vi "Periodic Tasks.vi"(8 "error in":errorcluster) -> ()   [LabVIEW 2014]
doc: "This VI runs in parallel to other tasks. It can contain as many user-defined periodic loops as you need. These can carry out PID or other sorts of timed response."
uses:
  <vilib>/Rock Robotics/WPI/Solenoid/WPI_SolenoidValue.ctl
  <vilib>/Rock Robotics/WPI/Joystick/WPI_JoystickGetSetRefNum.vi
  <vilib>/Rock Robotics/WPI/RobotDrive/WPI_RobotDriveGetSetRefNum.vi
  <vilib>/Rock Robotics/WPI/Solenoid/WPI_SolenoidSetEnum.vi
  <vilib>/Rock Robotics/WPI/Ultrasonic/WPI_UltrasonicRangeUnits.ctl
  <vilib>/Rock Robotics/WPI/Ultrasonic/WPI_SonarMB1010AnalogRefNum Registry Get.vi
panel:
  out "AVG Gyro Angle":dbl
  out "Gyro Angle 2":dbl
  out "error out":errorcluster
  out "Ultrasonic":i16
  out "USD Encoder":dbl
  out "limit switch":bool
  out "XY Graph 2":cluster{"Y":dbl[], "Y":dbl[]}[](graph)
  out "Accelerations":T1
  out "optical":bool
  out "potentiometer":dbl
  out "Gyro Angle":dbl
  out "Grayhill Encoder":dbl
  out "PDP voltage (V) IN":dbl
  in  "Value 2":T2
  in  "Value":T2
  in  "Output":dbl
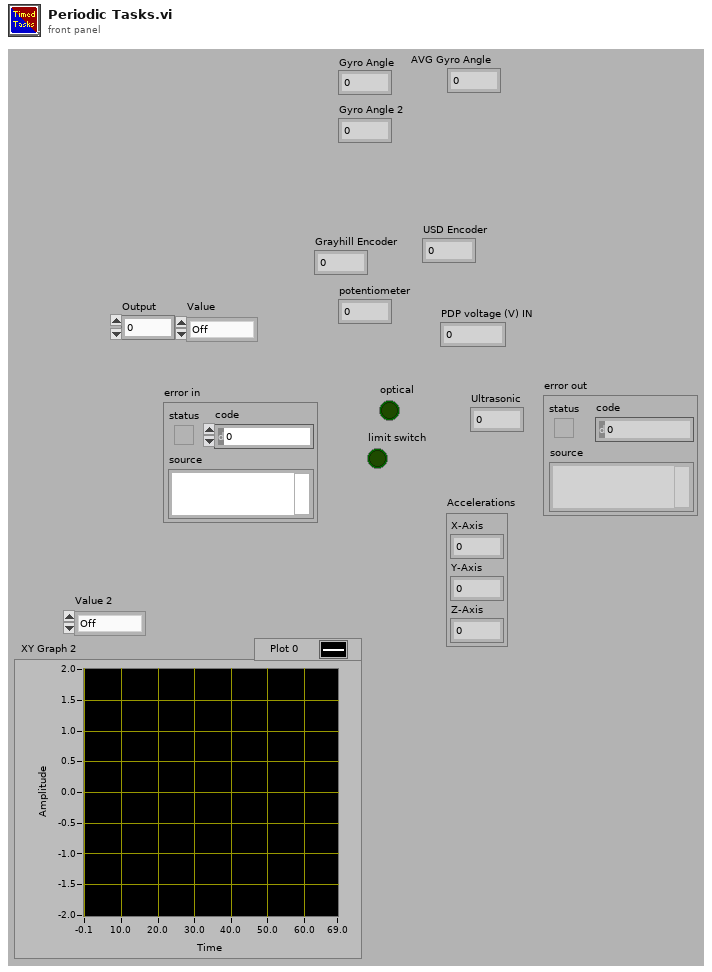
[diagram p1: front panel]
types:
  T1 = cluster{"X-Axis":dbl, "Y-Axis":dbl, "Z-Axis":dbl}
  T2 = typedef "WPI_SolenoidValue.ctl" = enum16{"Off", "On", "Forward", "Reverse"}
  T3 = typedef "WPI_CameraDevRef.ctl" = cluster{"Camera Address":string, "CameraStatus":errorcluster}
  T4 = typedef "WPI_JoystickDevRef.ctl" = cluster{"Device":T5}
  T5 = typedef "WPI_JoystickDeviceEnum.ctl" = enum16{"USB 0", "USB 1", "USB 2", "USB 3", "USB 4", "USB 5"}
  T6 = typedef "WPI_RobotDriveDevRef.ctl" = cluster{"DevStatus":errorcluster, "Motors[]":T7[], "Square Inputs":bool, "Max Output":dbl}
  T7 = typedef "WPI_MotorControlDeviceRef.ctl" = cluster{"DeviceStatus":errorcluster, "Type":T8, "PWM":cluster{"Controller":T9, "PWM Channel":T10, "DeadBand":T11}, "CAN":cluster{"Device Number":u8, "Control Mode":T12, "Semaphore":T13, "Max Vout":dbl, "TalonSRX Control Mode":T14}, "Invert":bool, "TransformRef":T15, "InvTransformRef":T15}
  T8 = typedef "WPI_MotorControlType.ctl" = enum16{"PWM", "CAN", "CANTalonSRX"}
  T9 = typedef "FPGA_TypedefDigitalModule.ctl" = enum16{"Controller 1"}
  T10 = typedef "FPGA_DIOPWMChannel.ctl" = enum8{"PWM 0", "PWM 1", "PWM 2", "PWM 3", "PWM 4", "PWM 5", "PWM 6", "PWM 7", "PWM 8", "PWM 9", "PWM MXP 0", "PWM MXP 1", "PWM MXP 2", "PWM MXP 3", "PWM MXP 4", "PWM MXP 5", "PWM MXP 6", "PWM MXP 7", "PWM MXP 8", "PWM MXP 9", "Invalid"}
  T11 = typedef "WPI_PWMDeadband.ctl" = cluster{"Name":string, "maxPositivePwm":i32, "minPositivePwm":i32, "centerPwm":i32, "maxNegativePwm":i32, "minNegativePwm":i32, "angularRange":u16}
  T12 = typedef "WPI_CANJaguar_ControlMode.ctl" = enum8{"Percent VBus", "Current", "Speed", "Position", "Voltage"}
  T13 = typedef "Semaphore RefNum" = refnum<k1>
  T14 = typedef "WPI_CANTalonSRX_APIControlMode.ctl" = enum8{"Percent VBus", "Speed", "Position", "Slave", "Unchanged / Invalid"}
  T15 = typedef "WPI_PWMTransform_ConPane.ctl" = refnum<vi>
  T16 = typedef "WPI_GyroDevRef.ctl" = cluster{"DevStatus":errorcluster, "Analog Module":T17, "Analog Channel":T18, "Offset":dbl, "Gain (VoltsPerDegree/Second)":dbl}
  T17 = typedef "FPGA_TypedefAnalogModule.ctl" = enum16{"Controller 1"}
  T18 = typedef "FPGA_AIChannel.ctl" = enum8{"AI 0", "AI 1", "AI 2", "AI 3", "AI MXP 0", "AI MXP 1", "AI MXP 2", "AI MXP 3", "Invalid"}
  T19 = cluster{"JoystickDevRef":T4, "RobotDriveDevRef":T6, "CameraDevRef":T3}
  T20 = typedef "WPI_EncoderDevRef.ctl" = cluster{"DevStatus":errorcluster, "EncoderIndex":T21, "CounterIndex":T22, "DistancePerCount":dbl, "Decoding Type":T23}
  T21 = typedef "FPGA_EncoderIdx.ctl" = enum8{"Enc 0", "Enc 1", "Enc 2", "Enc 3", "Enc 4", "Enc 5", "Enc 6", "Enc 7", "Invalid"}
  T22 = typedef "FPGA_CounterCtrSystemIndex.ctl" = enum8{"Ctr 0", "Ctr 1", "Ctr 2", "Ctr 3", "Ctr 4", "Ctr 5", "Ctr 6", "Ctr 7", "Invalid"}
  T23 = typedef "WPI_EncoderType.ctl" = enum16{"1x", "2x", "4x"}
  T24 = typedef "WPI_SwitchDevRef.ctl" = cluster{"DevStatus":errorcluster, "DIO Channel":T25, "Controller":T9, "CntIndex":T22, "Normally Closed":bool}
  T25 = typedef "FPGA_DIOChannel.ctl" = enum8{"DIO 0", "DIO 1", "DIO 2", "DIO 3", "DIO 4", "DIO 5", "DIO 6", "DIO 7", "DIO 8", "DIO 9", "DIO MXP 0", "DIO MXP 1", "DIO MXP 2", "DIO MXP 3", "DIO MXP 4", "DIO MXP 5", "DIO MXP 6", "DIO MXP 7", "DIO MXP 8", "DIO MXP 9", "DIO MXP 10", "DIO MXP 11", "DIO MXP 12", "DIO MXP 13", "DIO MXP 14", "DIO MXP 15", "Invalid"}
  T26 = typedef "WPI_PotentiometerDevRef.ctl" = cluster{"DevStatus":errorcluster, "Controller":T17, "Analog Channel":T18, "Invert Output":bool}
  T27 = typedef "WPI_AccelerometerDevRef.ctl" = cluster{"DevStatus":errorcluster, "Controller":T17, "Scaling":T28, "Analog Channels":T29, "I2C Bus":T30, "SPI Bus":T31, "Accel Range":T32, "ADXL345 Axes":T33, "Handle":i32, "Device Address":u8, "Accel Type":enum16{"Analog", "ADXL345 I2C", "ADXL345 SPI", "Internal"}}
  T28 = typedef "WPI_AccelerometerScaling.ctl" = cluster{"Gain (VoltsPerG)":dbl, "Center Voltage":dbl}
  T29 = typedef "WPI_AccelerometerAnalogChannels.ctl" = cluster{"X-Axis":T18, "Y-Axis":T18, "Z-Axis":T18}
  T30 = typedef "i2c_bus.ctl" = enum16{"I2C On-Board", "I2C MXP", "Invalid"}
  T31 = typedef "spi_bus.ctl" = enum16{"SPI On-Board, CS0", "SPI On-Board, CS1", "SPI On-Board, CS2", "SPI On-Board, CS3", "SPI MXP", "Invalid"}
  T32 = typedef "ADXL345 Range.ctl" = u8
  T33 = typedef "WPI_AccelerometerADXL345 Axes.ctl" = cluster{"X-Axis":bool, "Y-Axis":bool, "Z-Axis":bool}
  T34 = typedef "WPI_UltrasonicRangeUnits.ctl" = enum16{"inches", "mm"}
  T35 = typedef "WPI_AnalogChannelDevRef.ctl" = cluster{"DevStatus":errorcluster, "Controller":T17, "Analog Channel":T18}
  T36 = typedef "WPI_SolenoidDevRef.ctl" = cluster{"DevStatus":errorcluster, "Pneumatics Control Module":u8, "Forward Solenoid Channel":T37, "Reverse Solenoid Channel":T37}
  T37 = typedef "WPI_SolenoidChannel.ctl" = enum8{"Solenoid 0", "Solenoid 1", "Solenoid 2", "Solenoid 3", "Solenoid 4", "Solenoid 5", "Solenoid 6", "Solenoid 7", "Invalid"}
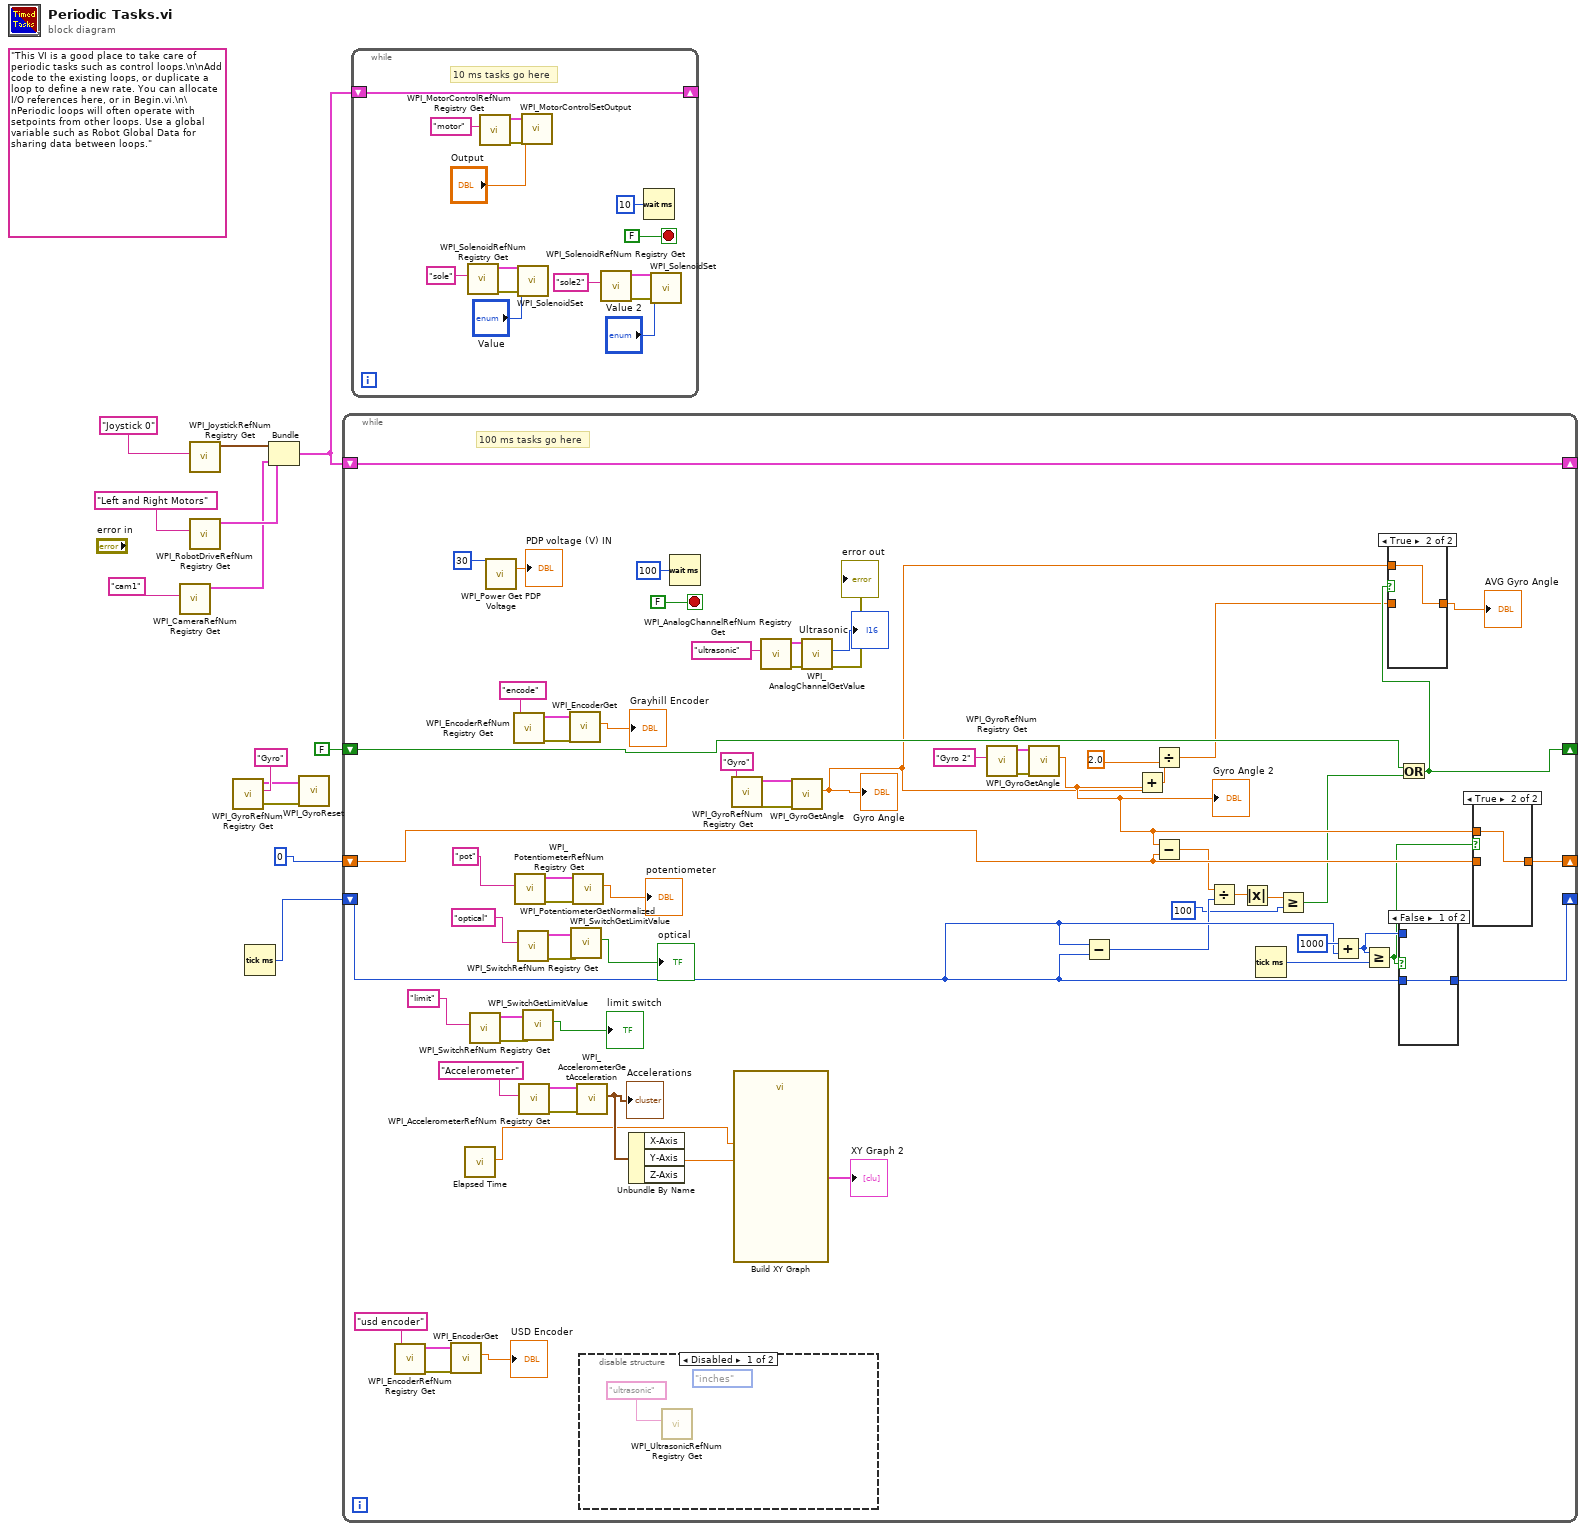
[diagram p0: block diagram]
diagram:
  (unwired) "This VI is a good place to take care of periodic tasks such as control loops.\n\nAdd code to the existing loops, or duplicate a loop to define a new rate. You can allocate I/O references here, or in Begin.vi.\n\nPeriodic loops will often operate with setpoints from other loops. Use a global variable such as Robot Global Data for sharing data between loops."
  n1 = call <vilib>:"WPI_CameraRefNum Registry Get.vi"("refnum name"="cam1") -> ("CameraDevRef"=w7:T3)  [unwired: 9 in, 1 out]
  n2 = call <vilib>:"WPI_JoystickRefNum Registry Get.vi"("refnum name"="Joystick 0") -> ("JoystickDevRef"=w11:T4)  [unwired: 1 in, 9 out]
  n3 = call <vilib>:"WPI_RobotDriveRefNum Registry Get.vi"("refnum name"="Left and Right Motors") -> ("RobotDriveDevRef"=w10:T6)  [unwired: 1 in, 9 out]
  n4 = call <vilib>:"WPI_GyroRefNum Registry Get.vi"("refnum name"="Gyro") -> ("error out"=w4:errorcluster, "GyroDevRef"=w5:T16)  [unwired: 9 in]
  n5 = Tick Count (ms)() -> (millisecond timer value=w3:u32)
  n6 = Bundle("JoystickDevRef"=w11, "RobotDriveDevRef"=w10, "CameraDevRef"=w7) -> (w9:T19)  [unwired: 1 out]
  n7 = call <vilib>:"WPI_GyroReset.vi"("error in (no error)"=w4, "GyroDevRef"=w5) -> ()  [unwired: 8 in, 2 out]
  n8 = while {
    shift-right: [w76] -> _
    shift-left: w9 -> [w76]
    shift-right: [w34] -> _
    shift-left: w3 -> [w28]
    shift-right: [w30] -> _
    shift-left: 0 -> [w26]
    shift-right: [w17] -> _
    shift-left: FALSE -> [w18]
    stop <- FALSE stop-if-true
    # "100 ms tasks go here"
    n9 = call <vilib>:"WPI_EncoderRefNum Registry Get.vi"("refnum name"="usd encoder") -> ("error out"=w46:errorcluster, "EncoderDevRef"=w47:T20)  [unwired: 9 in]
    n10 = call <vilib>:"WPI_EncoderGet.vi"("error in (no error)"=w46, "EncoderDevRef"=w47) -> ("Distance"=→"USD Encoder":dbl)  [unwired: 4 in, 5 out]
    n11 = call "Elapsed Time"() -> ("Elapsed Time (s)"=w52:dbl)  [unwired: 12 in, 7 out]
    n12 = call <vilib>:"WPI_SwitchRefNum Registry Get.vi"("refnum name"="limit") -> ("error out"=w51:errorcluster, "SwitchDevRef"=w50:T24)  [unwired: 9 in]
    n13 = call <vilib>:"WPI_Power Get PDP Voltage.vi"("Power Distribution Panel (0)"=30) -> ("voltage (V)"=→"PDP voltage (V) IN":dbl)  [unwired: 13 in, 1 out]
    n14 = call <vilib>:"WPI_EncoderRefNum Registry Get.vi"("refnum name"="encode") -> ("error out"=w72:errorcluster, "EncoderDevRef"=w73:T20)  [unwired: 9 in]
    n15 = call <vilib>:"WPI_PotentiometerRefNum Registry Get.vi"("refnum name"="pot") -> ("error out"=w65:errorcluster, "PotDevRef"=w66:T26)  [unwired: 9 in]
    n16 = call <vilib>:"WPI_SwitchRefNum Registry Get.vi"("refnum name"="optical") -> ("error out"=w62:errorcluster, "SwitchDevRef"=w61:T24)  [unwired: 9 in]
    n17 = call <vilib>:"WPI_AccelerometerRefNum Registry Get.vi"("refnum name"="Accelerometer") -> ("error out"=w58:errorcluster, "AccelerometerDevRef"=w57:T27)  [unwired: 9 in]
    n18 = call <vilib>:"WPI_SwitchGetLimitValue.vi"("error in (no error)"=w51, "SwitchDevRef"=w50) -> ("Switch Pressed"=→"limit switch":bool)  [unwired: 7 in, 2 out]
    n19 = call <vilib>:"WPI_EncoderGet.vi"("error in (no error)"=w72, "EncoderDevRef"=w73) -> ("Distance"=→"Grayhill Encoder":dbl)  [unwired: 4 in, 5 out]
    n20 = call <vilib>:"WPI_SwitchGetLimitValue.vi"("error in (no error)"=w62, "SwitchDevRef"=w61) -> ("Switch Pressed"=→"optical":bool)  [unwired: 7 in, 2 out]
    n21 = call <vilib>:"WPI_PotentiometerGetNormalized.vi"("error in"=w65, "PotDevRef"=w66) -> ("Normalized Value"=→"potentiometer":dbl)  [unwired: 7 in, 2 out]
    n22 = call <vilib>:"WPI_AccelerometerGetAcceleration.vi"("error in"=w58, "AccelerometerDevRef"=w57) -> ("Accelerations"=w53:T1)  [unwired: 7 in, 2 out]
    "Accelerations" <- w53
    n23 = disable-structure shown="Disabled" {
      frame Disabled {
        (unwired) WPI_UltrasonicRangeUnits."inches" ("Range Units")
        n24 = call-poly <vilib>:"WPI_UltrasonicRefNum Registry Get.vi"("refnum name"="ultrasonic") -> ()  [unwired: 9 in, 2 out]
      }
      frame Enabled {
      }
    }
    n25 = Unbundle By Name(w53) -> ("Y-Axis"=w54:dbl)  [unwired: 2 out]
    n26 = Wait (ms)(milliseconds to wait=u32 100) -> ()  [unwired: 1 out]
    n27 = call <vilib>:"WPI_GyroRefNum Registry Get.vi"("refnum name"="Gyro") -> ("error out"=w69:errorcluster, "GyroDevRef"=w70:T16)  [unwired: 9 in]
    n28 = call "Build XY Graph"("Y Input"=w54, "X Input"=w52) -> ("XY Graph"=→"XY Graph 2":cluster{"X":dbl[], "Y":dbl[]}[])  [unwired: 8 in, 1 out]
    n29 = call <vilib>:"WPI_AnalogChannelRefNum Registry Get.vi"("refnum name"="ultrasonic") -> ("error out"=w42:errorcluster, "AIDeviceRef"=w41:T35)  [unwired: 9 in]
    n30 = call <vilib>:"WPI_GyroGetAngle.vi"("error in (no error)"=w69, "GyroDevRef"=w70) -> ("Angle"=w14:dbl)  [unwired: 6 in, 3 out]
    "Gyro Angle" <- w14
    n31 = call <vilib>:"WPI_AnalogChannelGetValue.vi"("error in (no error)"=w42, "AIDeviceRef"=w41) -> ("error out"=→"error out":errorcluster, "Value"=→"Ultrasonic":i16)  [unwired: 7 in, 1 out]
    n32 = call <vilib>:"WPI_GyroRefNum Registry Get.vi"("refnum name"="Gyro 2") -> ("error out"=w37:errorcluster, "GyroDevRef"=w38:T16)  [unwired: 9 in]
    n33 = call <vilib>:"WPI_GyroGetAngle.vi"("error in (no error)"=w37, "GyroDevRef"=w38) -> ("Angle"=w27:dbl)  [unwired: 6 in, 3 out]
    "Gyro Angle 2" <- w27
    n34 = Subtract(x=w28, y=w28) -> (x-y=w24:u32)
    n35 = Add(x=w14, y=w27) -> (x+y=w29:dbl)
    n36 = Divide(x=w29, y=2.0) -> (x/y=w16:dbl)
    n37 = Subtract(x=w27, y=w26) -> (x-y=w25:dbl)
    n38 = Divide(x=w25, y=w24) -> (x/y=w23:dbl)
    n39 = Absolute Value(x=w23) -> (abs(x)=w22:dbl)
    n40 = Tick Count (ms)() -> (millisecond timer value=w33:u32)
    n41 = Greater Or Equal?(x=w22, y=100) -> (x >= y?=w19:bool)
    n42 = Add(x=1000, y=w28) -> (x+y=w31:u32)
    n43 = Greater Or Equal?(x=w31, y=w33) -> (x >= y?=w20:bool)
    n44 = Or(x=w18, y=w19) -> (x .or. y?=w17:bool)
    n45 = case shown="True" w17 {
      tunnel: w16 -> [w79 _]
      tunnel: [w79 w80] -> w15
      tunnel: w14 -> [_ w80]
      frame False {
      }
      frame True {
      }
    }
    "AVG Gyro Angle" <- w15
    n46 = case shown="False" w20 {
      tunnel: w28 -> [w83 _]
      tunnel: [w83 w84] -> w34
      tunnel: w31 -> [_ w84]
      frame False {
      }
      frame True {
      }
    }
    n47 = case shown="True" w20 {
      tunnel: w26 -> [w81 _]
      tunnel: [w81 w82] -> w30
      tunnel: w27 -> [_ w82]
      frame False {
      }
      frame True {
      }
    }
  }
  n48 = while {
    shift-right: [w98] -> _
    shift-left: w9 -> [w98]
    stop <- FALSE stop-if-true
    # "10 ms tasks go here"
    n49 = call <vilib>:"WPI_SolenoidRefNum Registry Get.vi"("refnum name"="sole") -> ("error out"=w93:errorcluster, "SolenoidDevRef"=w92:T36)  [unwired: 9 in]
    n50 = call <vilib>:"WPI_MotorControlRefNum Registry Get.vi"("refnum name"="motor") -> ("error out"=w97:errorcluster, "MotorControlDevRef"=w96:T7)  [unwired: 9 in]
    n51 = call-poly <vilib>:"WPI_SolenoidSet.vi"("error in (no error)"=w93, "Value"="Value", "SolenoidDevRef"=w92) -> ()  [unwired: 7 in, 2 out]
    n52 = call <vilib>:"WPI_MotorControlSetOutput.vi"("error in (no error)"=w97, "Output"="Output", "MotorControlDevRef"=w96) -> ()  [unwired: 6 in, 3 out]
    n53 = call <vilib>:"WPI_SolenoidRefNum Registry Get.vi"("refnum name"="sole2") -> ("error out"=w89:errorcluster, "SolenoidDevRef"=w88:T36)  [unwired: 9 in]
    n54 = Wait (ms)(milliseconds to wait=u32 10) -> ()  [unwired: 1 out]
    n55 = call-poly <vilib>:"WPI_SolenoidSet.vi"("error in (no error)"=w89, "Value"="Value 2", "SolenoidDevRef"=w88) -> ()  [unwired: 7 in, 2 out]
  }
